vi "LDH_automatisation_app.vi"() -> ()   [LabVIEW 2024]
panel:
  out "return value 2":dbl
  out "return value":dbl
  in  "write buffer 2":string
  out "return count 2":u32
  in  "byte count 2":u32
  out "read buffer 2":string
  in  "VISA resource name 2":refnum<visa-resource-name>
  out "Thermometer":dbl(slide) scale=-500.0..500.0
  out "Waveform Chart 2":dbl(graph)
  in  "Enum":T1(ring)=enum."Celsius [C]"
  out "Waveform Chart":cluster{dbl, "Numeric":dbl, dbl}[](graph)
  in  "Boolean":bool
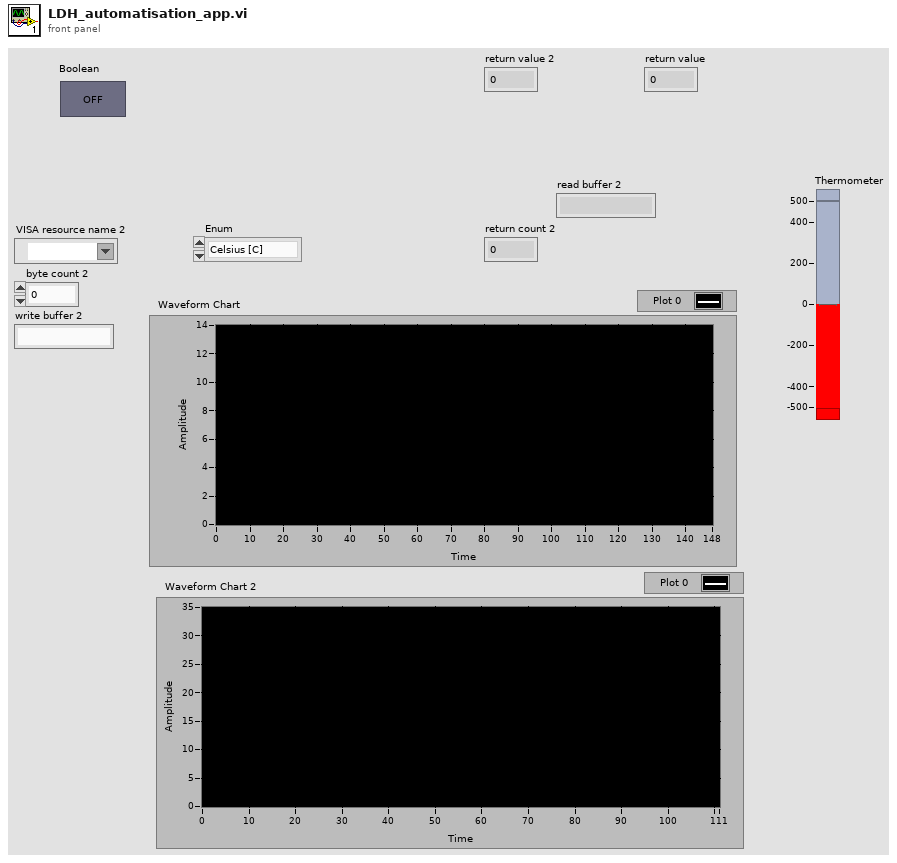
[diagram p1: front panel]
types:
  T1 = enum16{"Kelvin [K]", "Celsius [C]", "Fahrenheit [F]"}
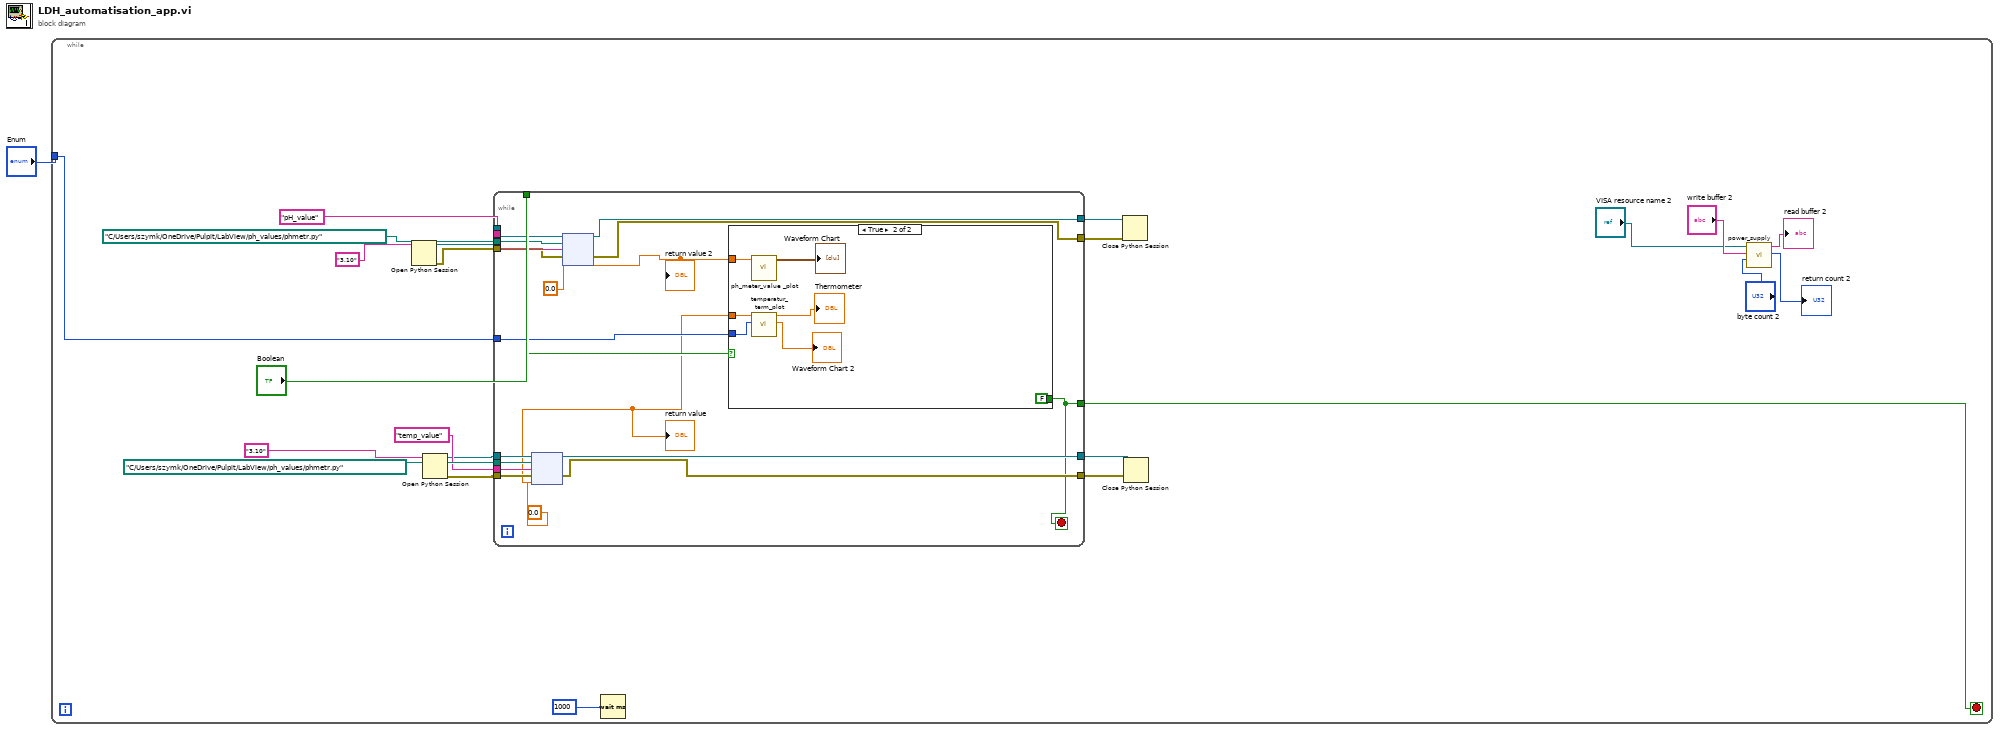
[diagram p0: block diagram]
diagram:
  n1 = while {
    tunnel: "Enum" -> [w10]
    stop <- w9 stop-if-true
    n2 = Open Python Session(python version="3.10" ("Python version")) -> (session out=w7:refnum<k35>, error out=w4:errorcluster)  [unwired: 2 in]
    n3 = Open Python Session(python version="3.10" ("Python version")) -> (session out=w13:refnum<k35>, error out=w12:errorcluster)  [unwired: 2 in]
    n4 = while {
      tunnel: w12 -> [w43]
      tunnel: w13 -> [w42]
      tunnel: "temp_value" -> [w41]
      tunnel: path "C:/Users/szymk/OneDrive/Pulpit/LabView/ph_values/phmetr.py" ("module path") -> [w40]
      tunnel: [w38] -> w17
      tunnel: [w37] -> w18
      tunnel: "Boolean" -> [w36]
      tunnel: w10 -> [w35]
      tunnel: [w34] -> w9
      tunnel: w7 -> [w32]
      tunnel: path "C:/Users/szymk/OneDrive/Pulpit/LabView/ph_values/phmetr.py" ("module path") -> [w31]
      tunnel: "pH_value" -> [w30]
      tunnel: w4 -> [w29]
      tunnel: [w27] -> w3
      tunnel: [w26] -> w2
      stop <- w34 stop-if-true
      n5 = node(w42, w40, w41, w43, 0.0) -> (w38:refnum<k35>, w37:errorcluster, w33:dbl)  [unwired: 2 out]
      "return value" <- w33
      n6 = node(w32, w31, w30, w29, 0.0) -> (w27:refnum<k35>, w26:errorcluster, w25:dbl)  [unwired: 2 out]
      "return value 2" <- w25
      n7 = case shown="True" w36 {
        selector: w36 -> [w44 _]
        tunnel: [w44 FALSE] -> w34
        tunnel: w33 -> [_ w47]
        tunnel: w35 -> [_ w46]
        tunnel: w25 -> [_ w45]
        frame False {
        }
        frame True {
          n8 = call "temperatur_term_plot.vi"("Enum"=w46, "Numeric in"=w47) -> ("Waveform Chart 2"=→"Waveform Chart 2":dbl, "Thermometer"=→"Thermometer":dbl)  [unwired: 8 in]
          n9 = call "ph_meter_value _plot.vi"("Numeric"=w45) -> ("Waveform Chart"=→"Waveform Chart":cluster{dbl, "Numeric":dbl, dbl}[])  [unwired: 10 in]
        }
      }
    }
    n10 = Wait (ms)(milliseconds to wait=1000) -> ()  [unwired: 1 out]
    n11 = Close Python Session(session in=w3, error in=w2) -> ()  [unwired: 1 out]
    n12 = Close Python Session(session in=w17, error in=w18) -> ()  [unwired: 1 out]
    n13 = call "power_supply.vi"("byte count in"="byte count 2", "write buffer in"="write buffer 2", "VISA Refnum in"="VISA resource name 2") -> ("return count 2"=→"return count 2":u32, "read buffer 2"=→"read buffer 2":string)  [unwired: 7 in]
  }
